vi "Tag Metadata Read Tags.vi"(0 "Path":path, 11 "Error In":errorcluster) -> (4 "Group Names":string[](array[string]), 6 "Tags":string[][](array[string]), 8 "Notes":string, 15 "Error Out":errorcluster)   [LabVIEW 2020]
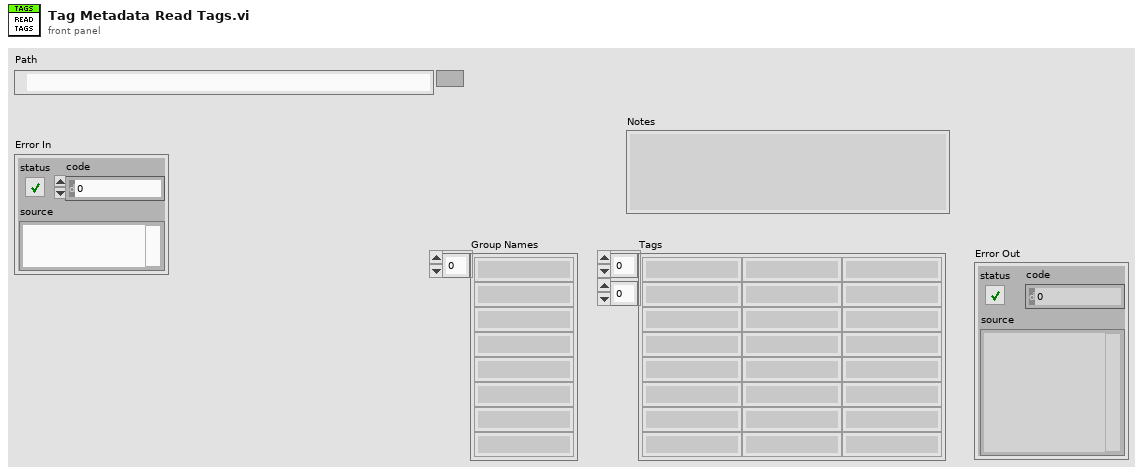
[diagram p1: front panel]
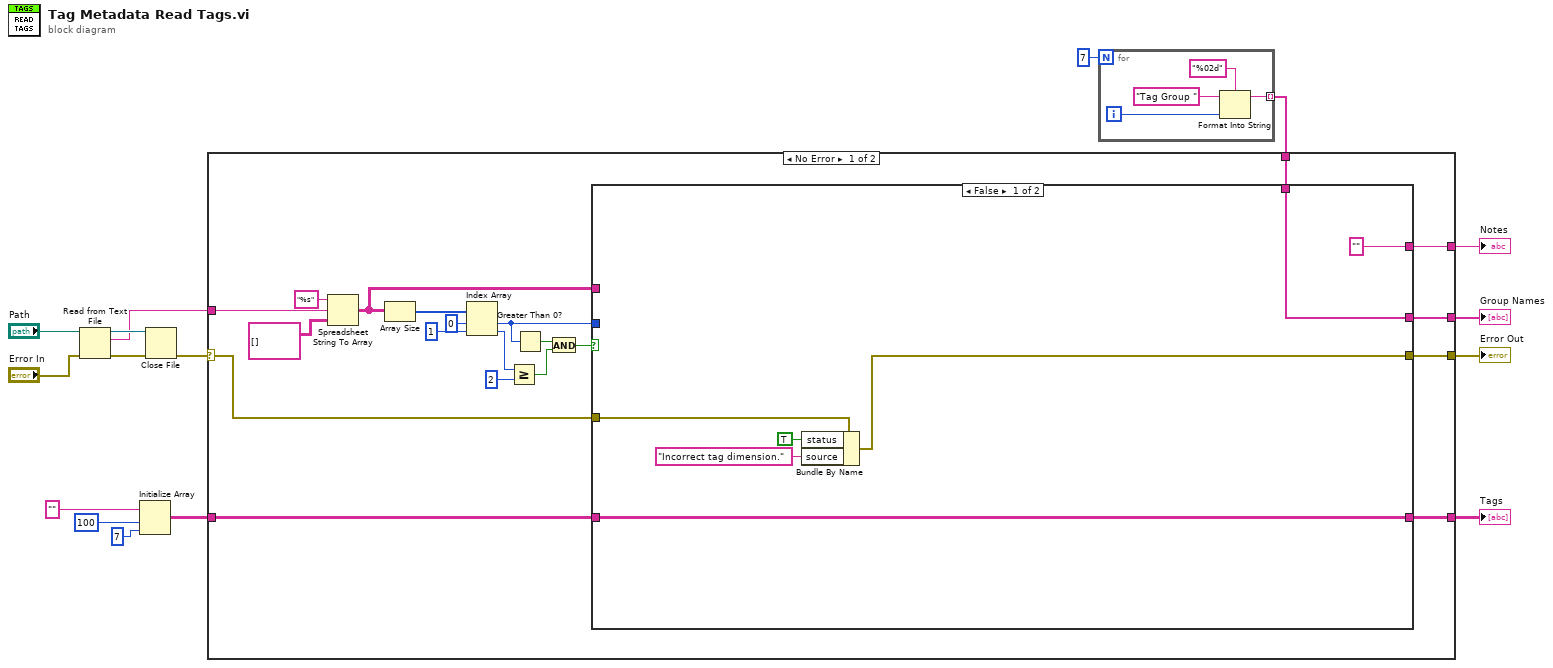
[diagram p0: block diagram]
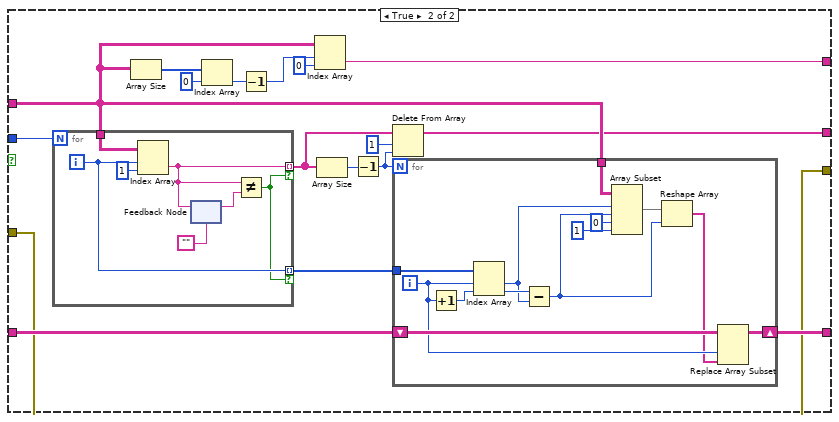
[diagram p2: hidden frame]
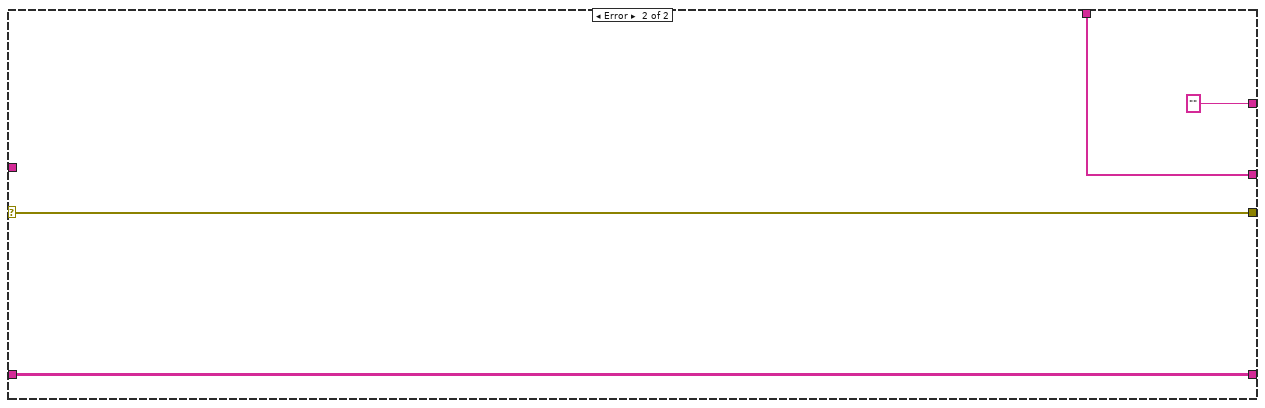
[diagram p3: hidden frame]
diagram:
  n1 = Read from Text File(file (use dialog)="Path", error in="Error In") -> (refnum out=w15:refnum<file>, text=w11:string, error out=w13:errorcluster)  [unwired: 2 in, 1 out]
  n2 = Initialize Array("", 100 ("dimension size"), 7 ("dimension size")) -> (w4:string[][])
  n3 = Close File(refnum=w15, error in=w13) -> (error out=w12:errorcluster)  [unwired: 1 out]
  n4 = for {
    N: 7 -> [_]
    tunnel: [w17] -> w3 mode=indexing
    i -> [w18]
    n5 = Format Into String(format string="%02d", initial string="Tag Group ", w18) -> (resulting string=w17:string)  [unwired: 1 in, 1 out]
  }
  n6 = case shown="No Error" w12 {
    selector: w12 -> [w22 w88]
    tunnel: w11 -> [w40 _]
    tunnel: [w21 w88] -> w2
    tunnel: [w27 w85] -> w10
    tunnel: [w26 w87] -> w9
    tunnel: [w25 ""] -> w8
    tunnel: w4 -> [w24 w85]
    tunnel: w3 -> [w23 w87]
    frame No Error {
      n7 = Spreadsheet String To Array(format string="%s", spreadsheet string=w40, array type (2D Dbl)=string[][] []) -> (array=w28:string[][])  [unwired: 1 in]
      n8 = Array Size(array=w28) -> (size(s)=w37:i32[])
      n9 = Index Array(array=w37, index #1=0 ("index"), index #2=1 ("index")) -> (element #1=w29:i32, element #2=w33:i32)
      n10 = Greater Or Equal?(x=w33, y=2) -> (x >= y?=w31:bool)
      n11 = Greater Than 0?(x=w29) -> (x > 0?=w34:bool)
      n12 = And(x=w34, y=w31) -> (x .and. y?=w30:bool)
      n13 = case shown="False" w30 {
        tunnel: w29 -> [_ w64]
        tunnel: w28 -> [_ w57]
        tunnel: w24 -> [w46 w61]
        tunnel: [w46 w60] -> w27
        tunnel: [w45 w51] -> w26
        tunnel: ["" w54] -> w25
        tunnel: w23 -> [w45 _]
        tunnel: w22 -> [w44 w48]
        tunnel: [w42 w48] -> w21
        frame False {
          n14 = Bundle By Name(cluster=w44, "status"=TRUE, "source"="Incorrect tag dimension.") -> (w42:errorcluster)
        }
        frame True {
          n15 = for {
            N: w64 -> [_]
            tunnel: [w81] -> w62 mode=indexing if=w79
            tunnel: [w80] -> w52 mode=indexing if=w79
            tunnel: w57 -> [w78]
            i -> [w81]
            n16 = Index Array(array=w78, index (row)=w81, index (col)=1 ("disabled index (col)")) -> (element=w80:string)
            n17 = feedback-in #1(w80) -> ()
            n18 = feedback #1("") -> (w83:string)
            n19 = Not Equal?(x=w80, y=w83) -> (x != y?=w79:bool)
          }
          n20 = Array Size(array=w57) -> (size(s)=w59:i32[])
          n21 = Index Array(array=w59, index=0) -> (element=w56:i32)
          n22 = Decrement(x=w56) -> (x-1=w53:i32)
          n23 = Index Array(array=w57, index (row)=w53, index (col)=0 ("disabled index (col)")) -> (element=w54:string)
          n24 = Array Size(array=w52) -> (size(s)=w63:i32)
          n25 = Decrement(x=w63) -> (x-1=w49:i32)
          n26 = Delete From Array(array=w52, length=1, index=w49) -> (array with subset deleted=w51:string[])  [unwired: 1 out]
          n27 = for {
            N: w49 -> [_]
            tunnel: w62 -> [w77]
            tunnel: w57 -> [w74]
            shift-right: [w65] -> w60
            shift-left: w61 -> [w68]
            i -> [w67]
            n28 = Increment(x=w67) -> (x+1=w76:i32)
            n29 = Index Array(array=w77, index #1=w67, index #2=w76) -> (element #1=w73:i32, element #2=w75:i32)
            n30 = Subtract(x=w75, y=w73) -> (x-y=w69:i32)
            n31 = Array Subset(array=w74, index (row)=w73, length (row)=w69, index (col)=0 ("index"), length (col)=1 ("length")) -> (w70:string[][])
            n32 = Reshape Array(w70, w69) -> (w66:string[])
            n33 = Replace Array Subset(array=w68, new element=w66, index (col)=w67) -> (w65:string[][])  [unwired: 1 in]
          }
        }
      }
    }
    frame Error {
    }
  }
  "Notes" <- w8
  "Group Names" <- w9
  "Tags" <- w10
  "Error Out" <- w2
